vi "Stop Core.vi"(10 "final error code":i32, 11 "Measurement in":refnum<class "Measurement.lvclass">) -> (3 "Measurement out":refnum<class "Measurement.lvclass">)   [LabVIEW 2017, in "Measurement Actor.lvlib" / "Measurement.lvclass"]
uses:
  Measurement.lvclass
  <vilib>/event_ctls.llb/usereventprio.ctl
  Measurement.lvclass/Measurement.ctl
  <vilib>/ActorFramework/Message Enqueuer/Message Enqueuer.lvclass/Message Enqueuer.ctl
  <vilib>/ActorFramework/Message Enqueuer/Enqueue.vi
  <vilib>/ActorFramework/Stop Msg/Stop Msg.lvclass
  C:/Program Files (x86)/National Instruments/LabVIEW 2017/vi.lib/ActorFramework/Message/Message.lvclass
  <vilib>/ActorFramework/Message Priority Queue/Priority Enqueue.vi
  <vilib>/ActorFramework/Actor/Actor.lvclass
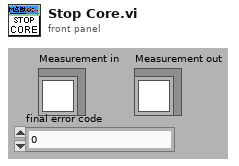
[diagram p1: front panel]
types:
  T1 = typedef "usereventprio.ctl" = enum32{"high priority", "normal priority"}
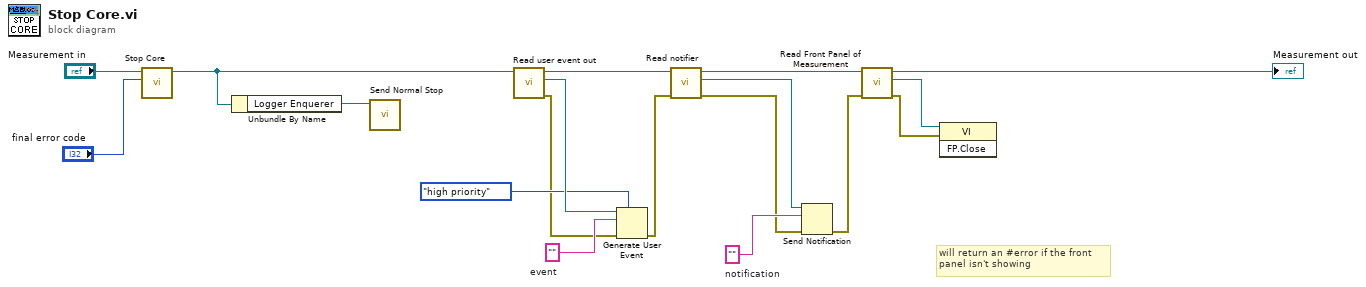
[diagram p0: block diagram]
diagram:
  w6 = ""  # event
  w16 = ""  # notification
  # "will return an #error if the front \npanel isn't showing"
  n1 = call-parent "Stop Core.vi"("final error code"="final error code", "Actor in"="Measurement in") -> ("Actor out"=w2:refnum<class "Measurement.lvclass">)  [unwired: 9 in]
  n2 = Unbundle By Name(w2) -> ("Logger Enquerer"=w1:refnum<class "Message Enqueuer.lvclass">)
  n3 = call <vilib>:"Send Normal Stop.vi"("Message Enqueuer"=w1) -> ()  [unwired: 10 in, 1 out]
  n4 = call "Read user event out.vi"("Measurement in"=w2) -> ("error out"=w5:errorcluster, "user event out"=w8:refnum<user-event>, "Measurement out"=w9:refnum<class "Measurement.lvclass">)  [unwired: 8 in]
  n5 = Generate User Event(priority (normal)=usereventprio."high priority", user event=w8, event data cluster=w6, error in=w5) -> (error out=w4:errorcluster)  [unwired: 1 out]
  n6 = call "Read notifier.vi"("error in (no error)"=w4, "Measurement in"=w9) -> ("error out"=w12:errorcluster, "notifier"=w17:refnum<notifier>, "Measurement out"=w13:refnum<class "Measurement.lvclass">)  [unwired: 7 in]
  n7 = Send Notification(notification=w16, notifier=w17, error in (no error)=w12) -> (error out=w11:errorcluster)  [unwired: 1 out]
  n8 = call "Read Front Panel of Measurement.vi"("error in (no error)"=w11, "Measurement in"=w13) -> ("error out"=w3:errorcluster, "Front Panel of Measurement"=w10:refnum<vi>, "Measurement out"=→"Measurement out":refnum<class "Measurement.lvclass">)  [unwired: 7 in]
  n9 = invoke class="VI" method="FP.Close"(reference=w10, error in=w3) -> ()  [unwired: 1 in, 3 out]
